vi "DateiZugriff.vi"() -> ()   [LabVIEW 2024]
panel:
  in  "StepSize":dbl max=0.0 step=10.0
  out "XY-Graph Z12":cluster{dbl[], i32[]}(graph)
  in  "Abbrechen":bool
  in  "Stop Value":dbl max=0.0 step=10.0
  out "Current Value":dbl
  in  "Start Value":dbl max=0.0 step=10.0
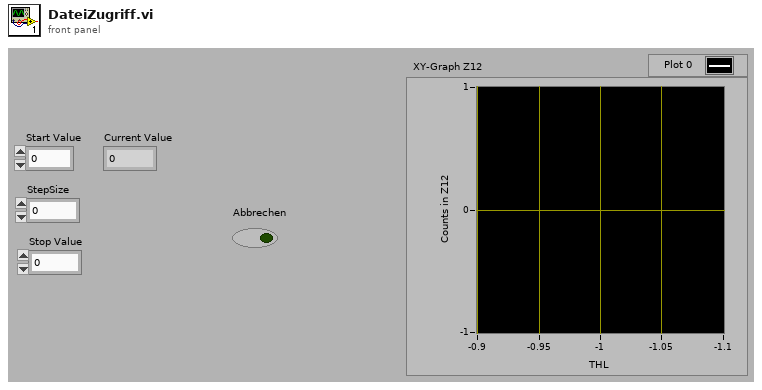
[diagram p1: front panel]
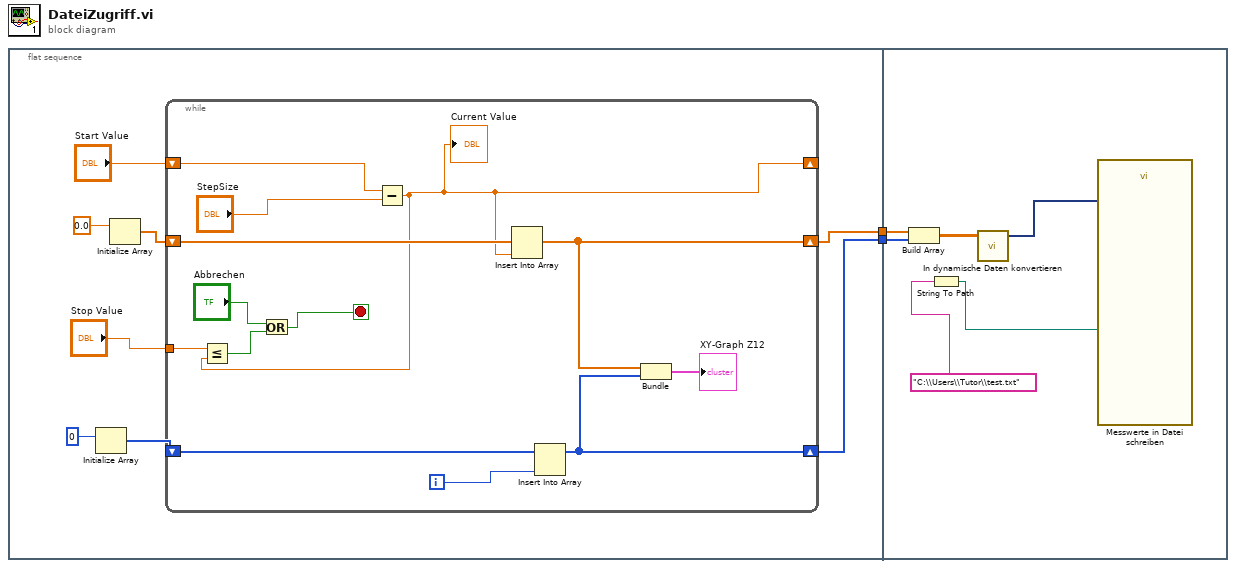
[diagram p0: block diagram]
diagram:
  n1 = flat-sequence {
    tunnel: [w7] -> w2
    tunnel: [w6] -> w1
    tunnel: w2 -> [w28]
    tunnel: w1 -> [w27]
    frame #0 {
      n2 = Initialize Array(0) -> (w9:i32[])  [unwired: 1 out]
      n3 = Initialize Array(0.0 ("Start Value 2")) -> (w4:dbl[])  [unwired: 1 out]
      n4 = while {
        shift-right: [w22] -> w7
        shift-left: w4 -> [w21]
        tunnel: "Stop Value" -> [w20]
        shift-right: [w17] -> w6
        shift-left: w9 -> [w23]
        shift-right: [w11] -> _
        shift-left: "Start Value" -> [w12]
        i -> [w16]
        stop <- w15 stop-if-true
        n5 = Subtract(x=w12, y="StepSize") -> (x-y=w11:dbl)
        "Current Value" <- w11
        n6 = Less Or Equal?(x=w20, y=w11) -> (x <= y?=w13:bool)
        n7 = Or(x="Abbrechen", y=w13) -> (x .or. y?=w15:bool)
        n8 = Insert Into Array(array=w21, new element=w11) -> (w22:dbl[])  [unwired: 1 in]
        n9 = Insert Into Array(array=w23, new element=w16) -> (w17:i32[])  [unwired: 1 in]
        n10 = Bundle(w22, w17) -> (→"XY-Graph Z12":cluster{dbl[], i32[]})  [unwired: 1 out]
      }
    }
    frame #1 {
      n11 = Build Array(w28, w27) -> (w25:dbl[][])
      n12 = String To Path(string="C:\\Users\\Tutor\\test.txt") -> (path=w24:path)
      n13 = call "In dynamische Daten konvertieren"("2D Array"=w25) -> ("Dynamic Data Type"=w29:dynamicdata)  [unwired: 3 out]
      n14 = call "Messwerte in Datei schreiben"("Signals"=w29, "Filename"=w24) -> ()  [unwired: 15 in, 3 out]
    }
  }
